vi "homework - wf chart with running average and fileIO.vi"() -> ()   [LabVIEW 2024]
doc: "#vi_description \nPlot a random number onto a waveform chart. Perform a running average of the most recent 4 points of data and store it to disk.\nThetic Engineering Ltd."
uses:
  <vilib>/Utility/sysdir.llb/System Directory Type.ctl
panel:
  in  "Record":bool
  in  "Stop":bool
  out "alarm":bool
  in  "threshold":dbl(knob)=0.49568843009143065 min=0.1 step=0.1 scale=0.1..0.9
  out "Waveform Chart":T1(graph)
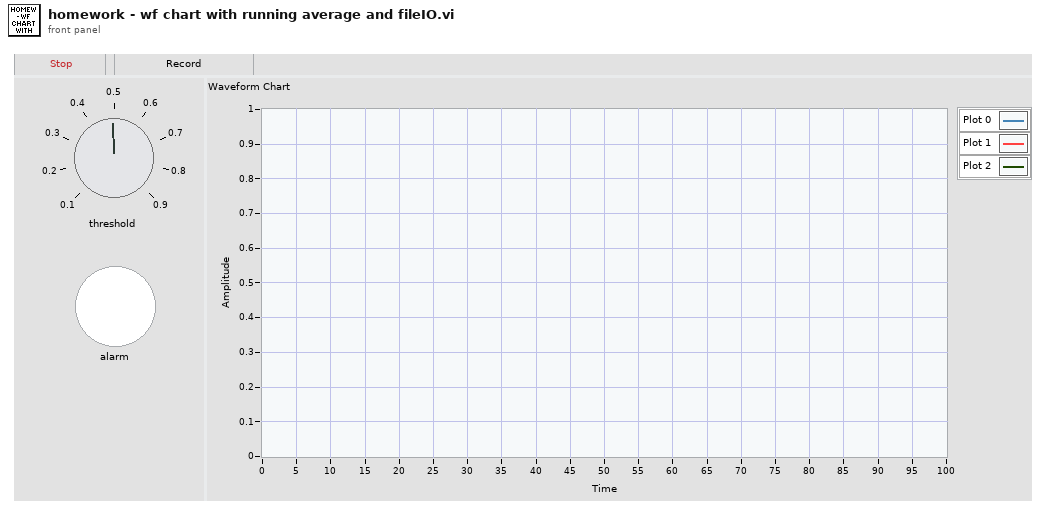
[diagram p1: front panel]
types:
  T1 = cluster{"number: 0 to 1":dbl, "threshold":dbl, dbl}
  T2 = enum16{"open", "replace", "create", "open or create", "replace or create", "replace or create with confirmation"}
  T3 = typedef "System Directory Type.ctl" = i32
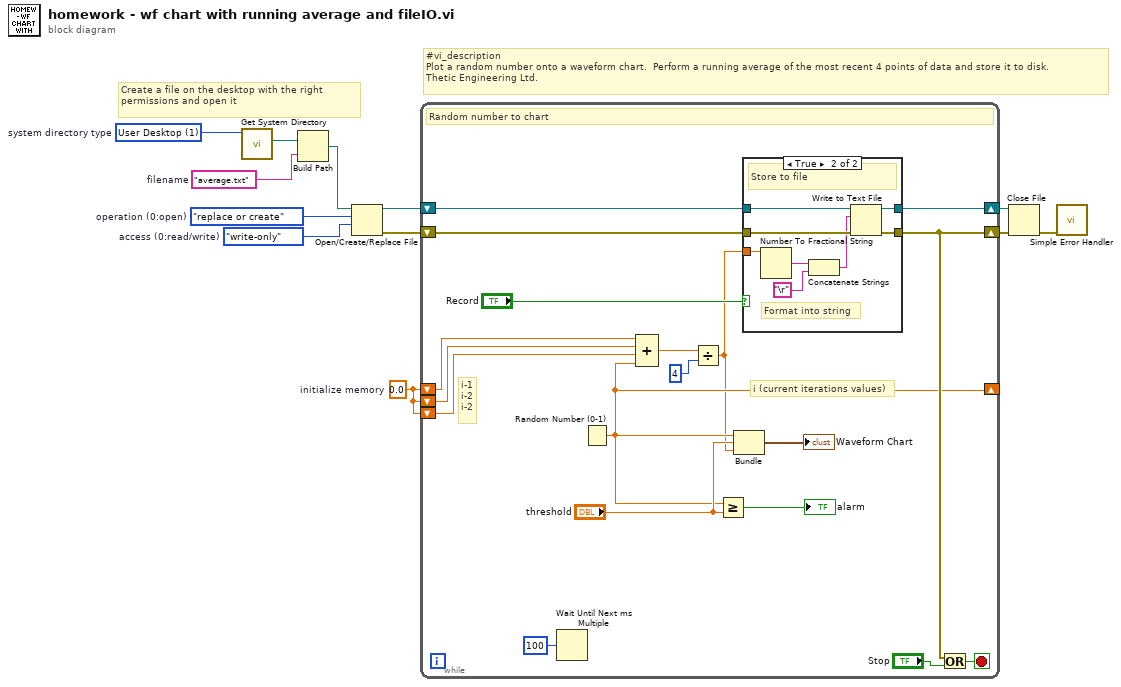
[diagram p0: block diagram]
diagram:
  w7 = "average.txt"  # filename
  w8 = enum16{"read/write", "read-only", "write-only"}."write-only"  # access (0:read/write)
  w9 = T2."replace or create"  # operation (0:open)
  w11 = T3 1 items=["User Home"=0, "User Desktop"=1, "User Documents"=2, "User Application Data"=3, "User Preferences"=4, "User Temporary"=5, "Public Documents"=6, "Public Application Data"=7, "Public Preferences"=8, "Public Cache"=13, "System Core Libraries"=9, "System Installed Libraries"=10, "Application Files"=11, "Boot Volume Root"=12]  # system directory type
  w12 = 0.0  # initialize memory
  # "Create a file on the desktop with the right permissions and open it"
  # "#vi_description \nPlot a random number onto a waveform chart.  Perform a running average of the most recent 4 points of data and store it to disk.\nThetic Engineering Ltd."
  n1 = call <vilib>:"Get System Directory.vi"("system directory type"=w11) -> ("system directory"=w10:path)  [unwired: 10 in]
  n2 = Build Path(base path=w10, name or relative path=w7) -> (appended path=w6:path)
  n3 = Open/Create/Replace File(file path (use dialog)=w6, operation (0:open)=w9, access (0:read/write)=w8) -> (refnum out=w4:refnum<file>, error out=w5:errorcluster)  [unwired: 3 in, 1 out]
  n4 = while {
    shift-right: [w24] -> _
    shift-left: w12 -> [w21]
    shift-left: w12 -> [w22]
    shift-left: w12 -> [w23]
    shift-right: [w15] -> w1
    shift-left: w4 -> [w17]
    shift-right: [w30] -> w2
    shift-left: w5 -> [w16]
    stop <- w13 stop-if-true
    # "i (current iterations values)"
    # "i-1\ni-2\ni-2"
    # "Random number to chart"
    n5 = Wait Until Next ms Multiple(millisecond multiple=u32 100) -> ()  [unwired: 1 out]
    n6 = Random Number (0-1)() -> (number: 0 to 1=w24:dbl)
    n7 = Compound Arithmetic op=ADD(w21, w22, w23, w24) -> (w20:dbl)
    n8 = Divide(x=w20, y=4) -> (x/y=w14:dbl)
    n9 = Greater Or Equal?(x=w24, y="threshold") -> (x >= y?=→"alarm":bool)
    n10 = Bundle("number: 0 to 1"=w24, "threshold"="threshold", w14) -> (→"Waveform Chart":T1)  [unwired: 1 in]
    n11 = case shown="True" "Record" {
      tunnel: w17 -> [w32 w38]
      tunnel: w16 -> [w31 w37]
      tunnel: [w32 w39] -> w15
      tunnel: [w31 w40] -> w30
      tunnel: w14 -> [_ w36]
      frame False {
        # "Do Nothing"
      }
      frame True {
        # "Format into string"
        # "Store to file"
        n12 = Number To Fractional String(number=w36) -> (F-format string=w35:string)  [unwired: 3 in]
        n13 = Concatenate Strings(w35, "\r") -> (w34:string)
        n14 = Write to Text File(file (use dialog)=w38, text=w34, error in=w37) -> (refnum out=w39:refnum<file>, error out=w40:errorcluster)  [unwired: 1 in, 1 out]
      }
    }
    n15 = Or(x=w30, y="Stop") -> (x .or. y?=w13:bool)
  }
  n16 = Close File(refnum=w1, error in=w2) -> (error out=w3:errorcluster)  [unwired: 1 out]
  n17 = call <vilib>:"Simple Error Handler.vi"("error in (no error)"=w3) -> ()  [unwired: 4 in, 5 out]
